vi "Is Open.vi"(8 "error in (no error)":errorcluster, 11 "Serial Client in":refnum<class "Serial Client.lvclass">) -> (0 "error out":errorcluster, 2 "Is Open":bool, 3 "Serial Client out":refnum<class "Serial Client.lvclass">)   [LabVIEW 2020, in "Stream-Serial.lvlib" / "Serial Client.lvclass"]
uses:
  Serial Client.lvclass
  lv-stream/stream/Connection/Connection.lvclass
  lv-stream/stream/Connection/State.ctl
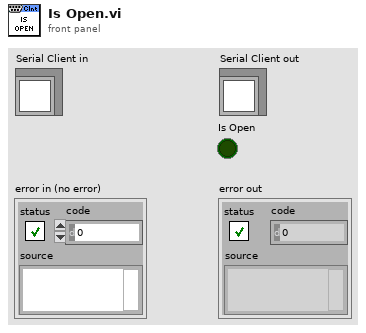
[diagram p1: front panel]
types:
  T1 = typedef "Stream.lvlib/Connection.lvclass/State.ctl" = enum16{"Closed", "Idle", "Connecting", "Connected", "Shutdown"}
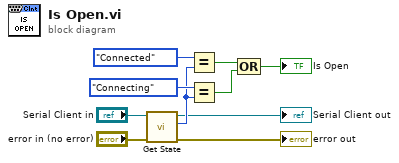
[diagram p0: block diagram]
diagram:
  n1 = call "Get State.vi"("error in (no error)"="error in (no error)", "Connection in"="Serial Client in") -> ("error out"=→"error out":errorcluster, "State"=w6:T1, "Connection out"=→"Serial Client out":refnum<class "Serial Client.lvclass">)  [unwired: 7 in]
  n2 = Equal?(x=State."Connected", y=w6) -> (x = y?=w5:bool)
  n3 = Equal?(x=State."Connecting", y=w6) -> (x = y?=w4:bool)
  n4 = Compound Arithmetic op=OR(w5, w4) -> (→"Is Open":bool)
